vi "Release.vi"(13 "Circuit cluster in":T1) -> ()   [LabVIEW 2016]
uses:
  TypeDefs/Circuit Cluster.ctl
  Classes/GateAbst/GateAbst.lvclass
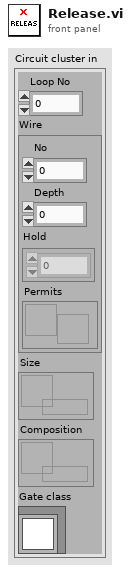
[diagram p1: front panel]
types:
  T1 = typedef "Circuit Cluster.ctl" = cluster{"Loop No":i32, "Wire":cluster{"No":i32, "Depth":i32, "Hold":i32[][], "Permits":refnum<notifier>}, "Size":refnum<queue>, "Composition":refnum<queue>, "Gate class":refnum<class "GateAbst.lvclass">}
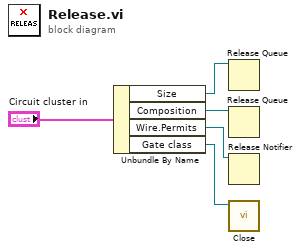
[diagram p0: block diagram]
diagram:
  n1 = Unbundle By Name("Circuit cluster in") -> ("Size"=w2:refnum<queue>, "Composition"=w3:refnum<queue>, "Wire.Permits"=w4:refnum<notifier>, "Gate class"=w5:refnum<class "GateAbst.lvclass">)
  n2 = Release Queue(queue=w2) -> ()  [unwired: 2 in, 3 out]
  n3 = Release Queue(queue=w3) -> ()  [unwired: 2 in, 3 out]
  n4 = Release Notifier(notifier=w4) -> ()  [unwired: 2 in, 3 out]
  n5 = call-dynamic "Close.vi"("GateAbst in"=w5) -> ()  [unwired: 9 in, 2 out]
